vi "Set up VICI.vi"() -> ()   [LabVIEW 2018]
uses:
  <vilib>/Instr/_visa.llb/VISA Configure Serial Port (Instr).vi
panel:
  in  "stop":bool
  out "read buffer 4":string
  out "Bytes at Port 5":u32
  out "read buffer 3":string
  out "Bytes at Port 4":u32
  out "String 2":string
  in  "Enum":enum16{"Enter", "Ctrl+J"}(ring)=enum."Ctrl+J"
  in  "message":string
  out "error out":errorcluster
  out "VISA resource name out":refnum<visa-resource-name>
  in  "VISA resource name":refnum<visa-resource-name>
  in  "error in (no error)":errorcluster
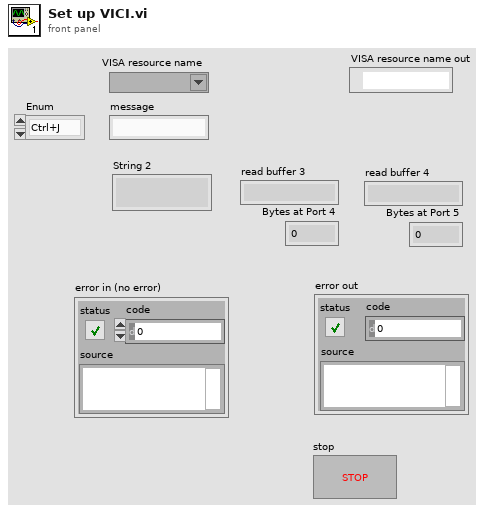
[diagram p1: front panel]
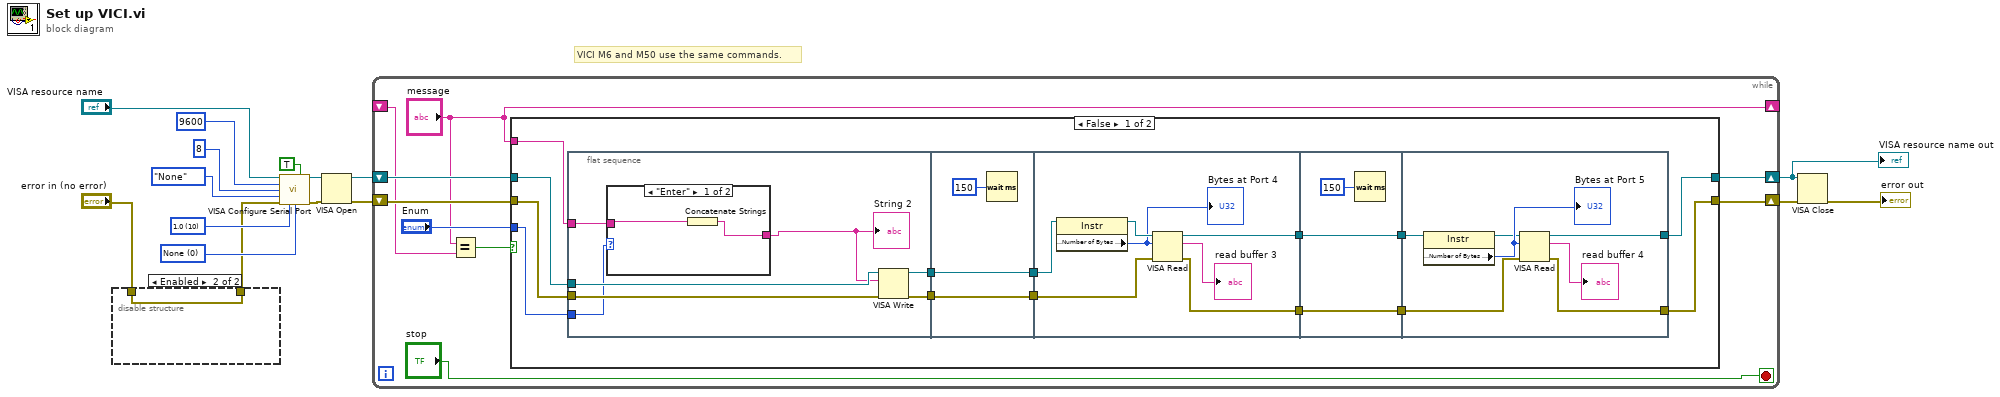
[diagram p0: block diagram]
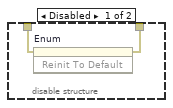
[diagram p2: hidden frame]
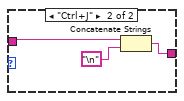
[diagram p3: hidden frame]
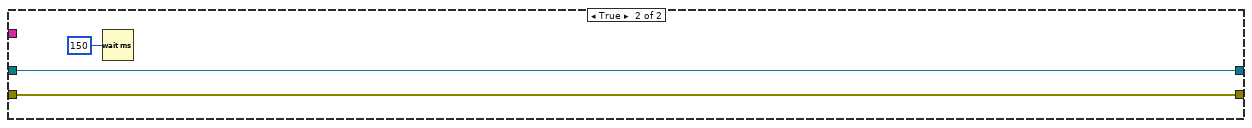
[diagram p4: hidden frame]
diagram:
  w9 = u16 0 items=["None", "XON/XOFF", "RTS/CTS", "XON/XOFF & RTS/CTS", "DTR/DSR", "XON/XOFF & DTR/DSR"] ("flow control (0:none)")
  w10 = u16 10 items=["1.0"=10, "1.5"=15, "2.0"=20] ("stop bits (10: 1 bit)")
  # "VICI M6 and M50 use the same commands."
  n1 = disable-structure shown="Enabled" {
    disable-tunnel: "error in (no error)" -> [w18 w19]
    disable-tunnel: [w17 w19] -> w2
    frame Disabled {
      n2 = invoke on="Enum" class="Enum (strict)" method="Reinit To Default"(error in=w18) -> (error out=w17:errorcluster)  [unwired: 2 in, 2 out]
    }
    frame Enabled {
    }
  }
  n3 = call-poly "VISA Configure Serial Port"("VISA resource name"="VISA resource name", "Enable Termination\nChar (T)"=TRUE ("Enable Termination\nChar (T)"), "baud rate (9600)"=u32 9600, "data bits (8)"=u16 8, "parity (0:none)"=enum16{"None", "Odd", "Even", "Mark", "Space"}."None", "error in (no error)"=w2, "stop bits (10: 1 bit)"=w10, "flow control (0:none)"=w9) -> ("VISA resource name out"=w15:refnum<visa-resource-name>, "error out"=w14:errorcluster)  [unwired: 6 in]
  n4 = VISA Open(error in (no error)=w14, VISA resource name=w15) -> (VISA resource name=w7:refnum<visa-resource-name>, error out=w8:errorcluster)  [unwired: 3 in]
  n5 = while {
    shift-right: [w26] -> w5
    shift-left: w8 -> [w28]
    shift-right: [w25] -> w4
    shift-left: w7 -> [w27]
    shift-right: ["message"] -> _
    shift-left: _ -> [w21]
    stop <- "stop" stop-if-true
    n6 = Equal?(x="message", y=w21) -> (x = y?=w23:bool)
    n7 = case shown="False" w23 {
      tunnel: w28 -> [w34 w75]
      tunnel: w27 -> [w33 w76]
      tunnel: "message" -> [w32 _]
      tunnel: [w31 w75] -> w26
      tunnel: [w30 w76] -> w25
      tunnel: "Enum" -> [w29 _]
      frame False {
        n8 = flat-sequence {
          tunnel: w33 -> [w49]
          tunnel: w32 -> [w48]
          tunnel: w34 -> [w47]
          tunnel: [w46] -> w42
          tunnel: [w45] -> w41
          tunnel: w29 -> [w43]
          tunnel: [w57] -> w40
          tunnel: w42 -> [w57]
          tunnel: [w56] -> w39
          tunnel: w41 -> [w56]
          tunnel: w40 -> [w61]
          tunnel: w39 -> [w60]
          tunnel: [w59] -> w38
          tunnel: [w58] -> w37
          tunnel: w38 -> [w67]
          tunnel: [w67] -> w36
          tunnel: w37 -> [w66]
          tunnel: [w66] -> w35
          tunnel: w36 -> [w71]
          tunnel: w35 -> [w70]
          tunnel: [w69] -> w30
          tunnel: [w68] -> w31
          frame #0 {
            n9 = case shown="\"Enter\"" w43 {
              tunnel: w48 -> [w51 w54]
              tunnel: [w50 w53] -> w44
              frame "Enter" {
                n10 = Concatenate Strings(w51) -> (w50:string)
              }
              frame "Ctrl+J" {
                n11 = Concatenate Strings(w54, "\n") -> (w53:string)
              }
            }
            "String 2" <- w44
            n12 = VISA Write(VISA resource name=w49, write buffer=w44, error in (no error)=w47) -> (VISA resource name out=w46:refnum<visa-resource-name>, error out=w45:errorcluster)  [unwired: 1 out]
          }
          frame #1 {
            n13 = Wait (ms)(milliseconds to wait=u32 150) -> ()  [unwired: 1 out]
          }
          frame #2 {
            n14 = property class="Instr"(reference=w61) -> (reference out=w64:refnum<visa-resource-name>, "Serial Settings:Number of Bytes at Serial Port"=w63:u32)  [unwired: 1 in, 1 out]
            "Bytes at Port 4" <- w63
            n15 = VISA Read(VISA resource name=w64, byte count=w63, error in (no error)=w60) -> (VISA resource name out=w59:refnum<visa-resource-name>, read buffer=→"read buffer 3":string, error out=w58:errorcluster)  [unwired: 1 out]
          }
          frame #3 {
            n16 = Wait (ms)(milliseconds to wait=u32 150) -> ()  [unwired: 1 out]
          }
          frame #4 {
            n17 = property class="Instr"(reference=w71) -> (reference out=w72:refnum<visa-resource-name>, "Serial Settings:Number of Bytes at Serial Port"=w73:u32)  [unwired: 1 in, 1 out]
            "Bytes at Port 5" <- w73
            n18 = VISA Read(VISA resource name=w72, byte count=w73, error in (no error)=w70) -> (VISA resource name out=w69:refnum<visa-resource-name>, read buffer=→"read buffer 4":string, error out=w68:errorcluster)  [unwired: 1 out]
          }
        }
      }
      frame True {
        n19 = Wait (ms)(milliseconds to wait=u32 150) -> ()  [unwired: 1 out]
      }
    }
  }
  "VISA resource name out" <- w4
  n20 = VISA Close(VISA resource name=w4, error in (no error)=w5) -> (error out=→"error out":errorcluster)
